vi "Create Plot.vi"(1 "clsData":T1) -> (0 "Plot":dbl[](array[numeric]))   [LabVIEW 2013]
doc: "This VI will create an xy plot based on the inputs m, b and Size according to the formula y=m*x+b"
uses:
  controls/clsData.ctl
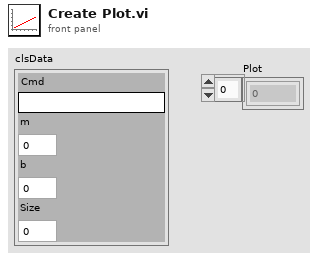
[diagram p1: front panel]
types:
  T1 = typedef "clsData.ctl" = cluster{"Cmd":string, "m":dbl, "b":dbl, "Size":u32}
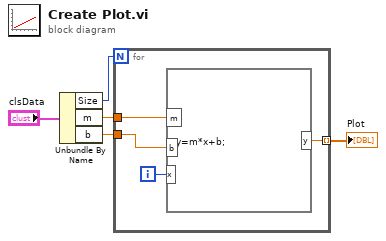
[diagram p0: block diagram]
diagram:
  n1 = Unbundle By Name("clsData") -> ("Size"=w4:u32, "m"=w3:dbl, "b"=w2:dbl)
  n2 = for {
    N: w4 -> [_]
    tunnel: w3 -> [w9]
    tunnel: w2 -> [w8]
    tunnel: [w6] -> w1 mode=indexing
    i -> [w7]
    n3 = formula code="y=m*x+b;"("m"=w9, "b"=w8, "x"=w7) -> ("y"=w6:dbl)
  }
  "Plot" <- w1
